vi "poly_h5_write_array_2d_DBL.vi"(0 "h5 dir ref":i32, 1 "dataset name":string, 5 "array":dbl[][](array[numeric]), 7 "units (au)":string="au", 11 "error in (no error)":errorcluster, 12 "dim1 (index)":string="index", 13 "dim2 (index)":string="index") -> (4 "h5 obj ref":i32, 15 "error out":errorcluster)   [LabVIEW 2015]
uses:
  <vilib>/addons/h5labview2/base/lib_path.vi
  <vilib>/addons/h5labview2/base/H5Equery.vi
  <vilib>/addons/h5labview2/dataset/H5Dwrite.llb/H5Dwrite.xnode
panel:
  # "Dim1 is the most recently added dimention. In general, DimN is changing faster the larger the N - C convention. - MK"
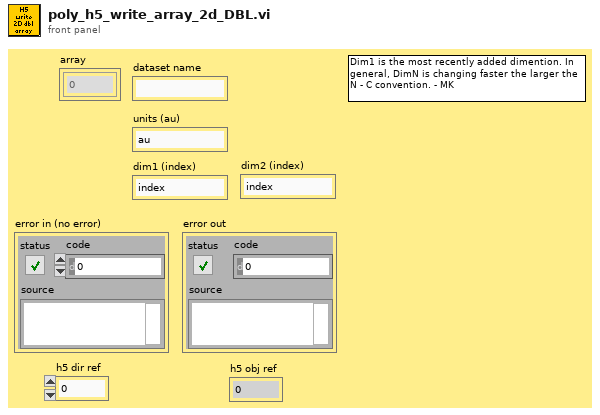
[diagram p1: front panel]
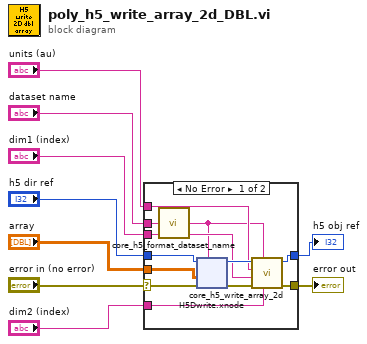
[diagram p0: block diagram]
diagram:
  n1 = case shown="No Error" "error in (no error)" {
    selector: "error in (no error)" -> [w19 w42]
    tunnel: "h5 dir ref" -> [w21 w41]
    tunnel: "units (au)" -> [w14 _]
    tunnel: "array" -> [w20 _]
    tunnel: "dataset name" -> [w11 _]
    tunnel: [w15 w42] -> w7
    tunnel: [w17 w41] -> w6
    tunnel: "dim1 (index)" -> [w13 _]
    tunnel: "dim2 (index)" -> [w12 _]
    frame No Error {
      n2 = call "core_h5_format_dataset_name.vi"("dataset name in"=w11) -> ("dataset name out"=w10:string)  [unwired: 8 in]
      n3 = xnode "H5Dwrite.xnode"("dataset name"=w10, "error in (no error)"=w19, "data"=w20, "ref in"=w21) -> ("error out"=w16:errorcluster, "ref out"=w18:i32)  [unwired: 3 in, 1 out]
      n4 = call "core_h5_write_array_2d.vi"("dim2 (index)"=w12, "dataset name"=w10, "error in (no error)"=w16, "dim1 (index)"=w13, "units (au)"=w14, "h5 obj ref"=w18) -> ("error out"=w15:errorcluster, "h5 obj ref"=w17:i32)  [unwired: 4 in]
    }
    frame Error {
    }
  }
  "error out" <- w7
  "h5 obj ref" <- w6
